vi "Parse.vi"(8 "Error In":errorcluster, 11 "object in":refnum<class "2024_5.lvclass">) -> (0 "Error Out":errorcluster, 3 "object out":refnum<class "2024_5.lvclass">)   [LabVIEW 2023, in "2024_5.lvclass"]
uses:
  2024_5.lvclass
  2024_5.lvclass/2024_5.ctl
  <vilib>/Utility/error.llb/Trim Whitespace One-Sided.vi
  <userlib>/_OpenG.lib/string/string.llb/openg_string.lvlib
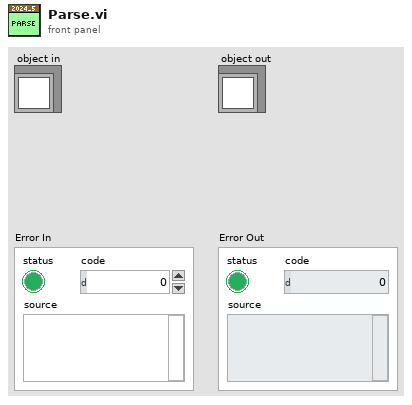
[diagram p1: front panel]
types:
  T1 = cluster{"default value 1":i64, "default value 1":i64}
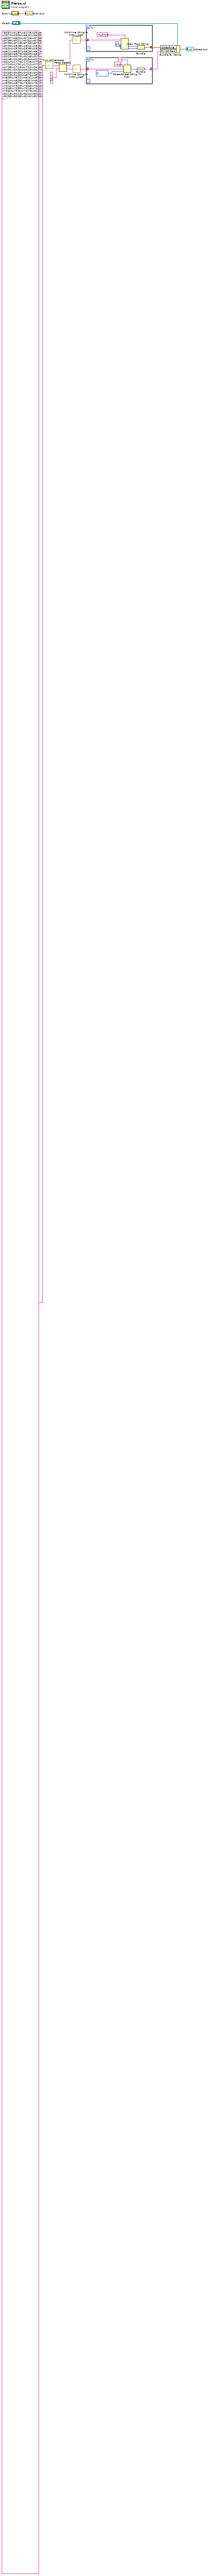
[diagram p0: block diagram]
diagram:
  n1 = call <vilib>:"Trim Whitespace.vi"("string"="39|57\n31|97\n31|75\n29|45\n29|73\n29|84\n66|91\n66|39\n66|57\n66|54\n97|16\n97|38\n97|59\n97|11\n97|62\n87|38\n87|59\n87|18\n87|93\n87|13\n87|33\n25|55\n25|22\n25|31\n25|64\n25|33\n25|85\n25|93\n68|11\n68|57\n68|36\n68|78\n68|66\n68|73\n68|39\n68|27\n32|29\n32|73\n32|45\n32|14\n32|48\n32|39\n32|54\n32|74\n32|17\n17|76\n17|45\n17|25\n17|14\n17|91\n17|11\n17|27\n17|38\n17|16\n17|22\n34|66\n34|91\n34|64\n34|29\n34|74\n34|65\n34|68\n34|26\n34|36\n34|13\n34|93\n48|76\n48|34\n48|55\n48|22\n48|42\n48|89\n48|14\n48|85\n48|87\n48|23\n48|38\n48|79\n73|62\n73|13\n73|42\n73|25\n73|55\n73|26\n73|65\n73|59\n73|18\n73|21\n73|64\n73|34\n73|79\n52|21\n52|18\n52|13\n52|22\n52|32\n52|55\n52|85\n52|42\n52|93\n52|39\n52|26\n52|66\n52|34\n52|68\n74|27\n74|57\n74|48\n74|73\n74|91\n74|16\n74|87\n74|38\n74|54\n74|75\n74|29\n74|62\n74|69\n74|84\n74|23\n38|37\n38|21\n38|13\n38|42\n38|64\n38|55\n38|66\n38|23\n38|85\n38|32\n38|79\n38|34\n38|89\n38|33\n38|52\n38|22\n69|65\n69|62\n69|38\n69|55\n69|34\n69|37\n69|33\n69|79\n69|21\n69|18\n69|87\n69|23\n69|85\n69|22\n69|16\n69|93\n69|89\n11|18\n11|85\n11|89\n11|59\n11|52\n11|22\n11|26\n11|87\n11|25\n11|76\n11|37\n11|23\n11|42\n11|21\n11|62\n11|38\n11|13\n11|69\n33|97\n33|27\n33|68\n33|29\n33|44\n33|31\n33|93\n33|66\n33|32\n33|84\n33|11\n33|45\n33|17\n33|54\n33|78\n33|75\n33|39\n33|36\n33|91\n91|79\n91|55\n91|22\n91|87\n91|23\n91|36\n91|25\n91|16\n91|76\n91|45\n91|59\n91|11\n91|75\n91|29\n91|62\n91|27\n91|69\n91|54\n91|48\n91|52\n75|34\n75|21\n75|42\n75|25\n75|76\n75|79\n75|23\n75|89\n75|18\n75|22\n75|26\n75|62\n75|69\n75|73\n75|11\n75|85\n75|37\n75|14\n75|52\n75|59\n75|38\n59|55\n59|13\n59|79\n59|32\n59|65\n59|93\n59|42\n59|52\n59|18\n59|44\n59|37\n59|85\n59|22\n59|25\n59|68\n59|33\n59|38\n59|31\n59|21\n59|23\n59|89\n59|26\n26|29\n26|39\n26|44\n26|31\n26|91\n26|17\n26|32\n26|93\n26|74\n26|66\n26|48\n26|57\n26|36\n26|97\n26|13\n26|45\n26|64\n26|65\n26|27\n26|33\n26|84\n26|78\n26|68\n79|42\n79|26\n79|57\n79|31\n79|89\n79|93\n79|18\n79|17\n79|33\n79|68\n79|74\n79|39\n79|85\n79|37\n79|78\n79|21\n79|44\n79|66\n79|65\n79|34\n79|64\n79|32\n79|97\n79|13\n42|37\n42|18\n42|13\n42|97\n42|29\n42|39\n42|78\n42|64\n42|65\n42|66\n42|89\n42|26\n42|44\n42|57\n42|85\n42|34\n42|32\n42|93\n42|31\n42|74\n42|91\n42|17\n42|33\n42|68\n18|17\n18|97\n18|44\n18|36\n18|29\n18|33\n18|91\n18|27\n18|64\n18|74\n18|57\n18|65\n18|13\n18|68\n18|84\n18|26\n18|78\n18|39\n18|66\n18|54\n18|93\n18|31\n18|32\n18|37\n22|26\n22|93\n22|13\n22|78\n22|66\n22|37\n22|31\n22|97\n22|34\n22|32\n22|85\n22|21\n22|39\n22|42\n22|65\n22|64\n22|44\n22|33\n22|89\n22|74\n22|79\n22|68\n22|55\n22|18\n62|44\n62|25\n62|85\n62|22\n62|64\n62|33\n62|13\n62|87\n62|26\n62|89\n62|16\n62|23\n62|79\n62|38\n62|59\n62|93\n62|55\n62|37\n62|18\n62|21\n62|42\n62|34\n62|65\n62|52\n21|34\n21|66\n21|93\n21|17\n21|44\n21|37\n21|68\n21|26\n21|74\n21|57\n21|18\n21|91\n21|65\n21|13\n21|31\n21|89\n21|32\n21|85\n21|39\n21|97\n21|78\n21|42\n21|64\n21|33\n93|84\n93|11\n93|57\n93|45\n93|36\n93|29\n93|76\n93|39\n93|31\n93|14\n93|91\n93|32\n93|66\n93|75\n93|48\n93|97\n93|78\n93|73\n93|74\n93|54\n93|17\n93|27\n93|44\n93|68\n23|32\n23|26\n23|68\n23|79\n23|39\n23|64\n23|25\n23|65\n23|22\n23|85\n23|31\n23|93\n23|55\n23|21\n23|13\n23|89\n23|37\n23|66\n23|52\n23|18\n23|33\n23|44\n23|42\n23|34\n84|52\n84|73\n84|11\n84|55\n84|14\n84|87\n84|76\n84|89\n84|16\n84|62\n84|48\n84|42\n84|54\n84|21\n84|69\n84|38\n84|22\n84|45\n84|79\n84|34\n84|23\n84|75\n84|59\n84|25\n16|22\n16|18\n16|85\n16|65\n16|37\n16|44\n16|13\n16|21\n16|38\n16|59\n16|25\n16|23\n16|87\n16|55\n16|68\n16|52\n16|89\n16|33\n16|34\n16|64\n16|42\n16|79\n16|26\n16|93\n85|44\n85|65\n85|39\n85|37\n85|84\n85|57\n85|64\n85|26\n85|32\n85|91\n85|74\n85|33\n85|18\n85|27\n85|78\n85|93\n85|17\n85|97\n85|66\n85|31\n85|36\n85|29\n85|13\n85|68\n55|26\n55|89\n55|64\n55|37\n55|78\n55|44\n55|93\n55|68\n55|39\n55|97\n55|79\n55|17\n55|21\n55|31\n55|85\n55|66\n55|13\n55|65\n55|42\n55|18\n55|34\n55|33\n55|32\n55|74\n65|75\n65|66\n65|11\n65|78\n65|39\n65|68\n65|44\n65|97\n65|36\n65|31\n65|45\n65|91\n65|14\n65|48\n65|33\n65|57\n65|84\n65|17\n65|93\n65|54\n65|27\n65|29\n65|74\n65|32\n76|37\n76|25\n76|42\n76|69\n76|23\n76|18\n76|16\n76|89\n76|62\n76|52\n76|34\n76|55\n76|21\n76|13\n76|79\n76|38\n76|65\n76|85\n76|26\n76|59\n76|87\n76|73\n76|64\n76|22\n27|21\n27|55\n27|38\n27|79\n27|59\n27|73\n27|75\n27|11\n27|16\n27|62\n27|42\n27|23\n27|76\n27|22\n27|45\n27|34\n27|52\n27|84\n27|87\n27|25\n27|48\n27|69\n27|54\n27|14\n14|52\n14|73\n14|22\n14|69\n14|25\n14|34\n14|16\n14|23\n14|21\n14|37\n14|38\n14|64\n14|87\n14|85\n14|59\n14|26\n14|13\n14|18\n14|76\n14|42\n14|62\n14|79\n14|55\n14|89\n36|48\n36|75\n36|23\n36|21\n36|73\n36|84\n36|54\n36|87\n36|25\n36|62\n36|42\n36|16\n36|79\n36|76\n36|27\n36|38\n36|11\n36|22\n36|69\n36|52\n36|45\n36|14\n36|55\n36|59\n13|17\n13|44\n13|27\n13|93\n13|32\n13|33\n13|66\n13|48\n13|91\n13|31\n13|54\n13|78\n13|57\n13|29\n13|64\n13|84\n13|74\n13|68\n13|39\n13|45\n13|97\n13|36\n13|75\n13|65\n57|29\n57|14\n57|54\n57|25\n57|76\n57|45\n57|59\n57|69\n57|91\n57|75\n57|87\n57|27\n57|16\n57|11\n57|22\n57|84\n57|55\n57|73\n57|38\n57|36\n57|48\n57|62\n57|52\n57|23\n89|29\n89|18\n89|66\n89|37\n89|33\n89|68\n89|39\n89|85\n89|13\n89|44\n89|97\n89|27\n89|91\n89|32\n89|93\n89|31\n89|64\n89|36\n89|74\n89|57\n89|17\n89|65\n89|26\n89|78\n78|75\n78|23\n78|45\n78|48\n78|69\n78|25\n78|17\n78|84\n78|73\n78|29\n78|36\n78|14\n78|91\n78|57\n78|76\n78|87\n78|62\n78|27\n78|38\n78|16\n78|11\n78|54\n78|59\n78|52\n64|33\n64|27\n64|44\n64|57\n64|78\n64|11\n64|65\n64|48\n64|31\n64|93\n64|39\n64|45\n64|17\n64|84\n64|91\n64|74\n64|29\n64|75\n64|68\n64|97\n64|32\n64|36\n64|54\n64|66\n54|34\n54|16\n54|79\n54|85\n54|23\n54|87\n54|69\n54|73\n54|52\n54|21\n54|14\n54|75\n54|22\n54|11\n54|48\n54|59\n54|25\n54|38\n54|45\n54|55\n54|89\n54|76\n54|62\n54|42\n37|91\n37|65\n37|44\n37|13\n37|31\n37|64\n37|17\n37|66\n37|33\n37|36\n37|78\n37|93\n37|68\n37|74\n37|32\n37|29\n37|26\n37|48\n37|39\n37|54\n37|97\n37|84\n37|57\n37|27\n44|54\n44|75\n44|68\n44|69\n44|14\n44|45\n44|97\n44|17\n44|84\n44|29\n44|74\n44|78\n44|27\n44|66\n44|31\n44|39\n44|32\n44|91\n44|57\n44|76\n44|11\n44|48\n44|73\n44|36\n45|76\n45|34\n45|73\n45|21\n45|85\n45|38\n45|59\n45|25\n45|79\n45|87\n45|11\n45|62\n45|52\n45|75\n45|16\n45|37\n45|18\n45|23\n45|22\n45|89\n45|69\n45|55\n45|42\n45|14\n39|29\n39|73\n39|48\n39|59\n39|38\n39|36\n39|87\n39|14\n39|54\n39|91\n39|17\n39|74\n39|76\n39|11\n39|62\n39|78\n39|16\n39|45\n39|69\n39|27\n39|75\n39|97\n39|84\n31|57\n31|48\n31|39\n31|11\n31|27\n31|74\n31|54\n31|66\n31|36\n31|91\n31|16\n31|78\n31|87\n31|45\n31|17\n31|76\n31|84\n31|69\n31|14\n31|29\n31|62\n31|73\n29|11\n29|87\n29|79\n29|25\n29|16\n29|36\n29|22\n29|48\n29|21\n29|62\n29|14\n29|69\n29|75\n29|55\n29|59\n29|76\n29|23\n29|52\n29|38\n29|27\n29|54\n66|14\n66|59\n66|69\n66|27\n66|75\n66|62\n66|84\n66|45\n66|17\n66|78\n66|76\n66|97\n66|87\n66|11\n66|16\n66|36\n66|73\n66|29\n66|48\n66|74\n97|27\n97|91\n97|29\n97|57\n97|78\n97|45\n97|54\n97|14\n97|48\n97|23\n97|69\n97|17\n97|36\n97|73\n97|74\n97|76\n97|84\n97|87\n97|75\n87|44\n87|85\n87|79\n87|55\n87|21\n87|23\n87|22\n87|65\n87|64\n87|42\n87|26\n87|68\n87|32\n87|52\n87|34\n87|89\n87|25\n87|37\n25|34\n25|21\n25|65\n25|42\n25|26\n25|13\n25|44\n25|79\n25|18\n25|68\n25|97\n25|89\n25|32\n25|37\n25|39\n25|74\n25|66\n68|32\n68|62\n68|45\n68|91\n68|29\n68|74\n68|54\n68|14\n68|69\n68|75\n68|84\n68|76\n68|17\n68|48\n68|97\n68|31\n32|69\n32|31\n32|11\n32|27\n32|66\n32|36\n32|97\n32|75\n32|76\n32|84\n32|91\n32|16\n32|57\n32|78\n32|62\n17|57\n17|23\n17|36\n17|69\n17|29\n17|73\n17|75\n17|62\n17|59\n17|48\n17|87\n17|84\n17|54\n17|52\n34|31\n34|57\n34|32\n34|85\n34|39\n34|37\n34|78\n34|17\n34|97\n34|44\n34|18\n34|89\n34|33\n48|52\n48|75\n48|21\n48|59\n48|18\n48|69\n48|73\n48|16\n48|62\n48|11\n48|45\n48|25\n73|52\n73|33\n73|16\n73|85\n73|89\n73|23\n73|87\n73|22\n73|38\n73|69\n73|37\n52|64\n52|31\n52|44\n52|33\n52|25\n52|97\n52|65\n52|89\n52|79\n52|37\n74|36\n74|76\n74|17\n74|11\n74|78\n74|14\n74|52\n74|45\n74|59\n38|26\n38|65\n38|31\n38|68\n38|93\n38|44\n38|25\n38|18\n69|13\n69|26\n69|25\n69|52\n69|42\n69|59\n69|64\n11|16\n11|73\n11|34\n11|55\n11|14\n11|79\n33|74\n33|14\n33|48\n33|76\n33|57\n91|14\n91|38\n91|73\n91|84\n75|55\n75|87\n75|16\n59|34\n59|64\n26|54\n\n78,45,48,38,52,62,29\n87,59,38,52,25,55,79,42,34,85,37,26,13,64,65,33,68\n57,29,84,48,45,75,11,14,76,73,69,16,38,23,22\n74,57,91,36,27,84,54,45,75,11,14,76,73,69,87,59,38\n69,62,16,87,59,38,23,52,25,22,55,79,21,42,34,89,85,18,37,26,13,64,33\n33,44,68,32,31,66,39,97,74,78,17,57,91,29,36,27,54,48,75,11,14\n32,66,39,97,74,78,17,57,91,29,36,27,84,54,48,45,11,14,73,69,62\n74,66,65,34,93,32,21,26,89,31,78,44,18,13,37,85,33,68,79,64,55\n38,52,25,55,21,34,85,18,26,13,64,33,93,44,68,32,31\n68,36,64,33,48,32,93,31,13,26,74\n48,45,75,11,76,73,69,62,87,59,38,23,22,55,79,21,42,34,85\n33,16,44,34,85,79,65,22,42,25,64,87,18,55,52,89,13\n73,69,62,16,87,59,38,23,52,25,22,55,79,21,42,89,85,18,37,26,13,64,65\n14,78,45,23,16,36,57,74,76,87,75,59,62,73,54,27,17,91,48,29,84,69,38\n33,93,44,32,31,66,97,74,78,17,57,91,29,36,84,54,48,45,75,11,14\n38,23,79,42,34,37,33,32,31\n65,93,44,68,32,31,66,39,97,74,78,17,57,91,36,27,84,54,48,75,11\n11,84,59,45,54,38,36,14,29,52,16,27,62,76,87,78,75\n54,48,45,75,11,14,76,73,69,62,16,87,59,38,23,52,25,22,55,79,21,34,89\n34,18,26,74,29,31,85,17,64\n16,87,38,52,21,34,18,37,13,64,33\n91,31,78,66,27,84,74,36,32,39,68,73,44\n69,62,36,74,45,66,54,91,14,11,27,32,75,39,84,48,73,76,31,29,17,78,97\n44,68,32,31,66,74,78,57,36,27,84,54,14,76,73\n59,73,22,21,76,62,14,23,16,79,27,36,55,75,38,54,48,11,52,45,25,84,69\n29,36,27,54,45,75,11,14,73,69,62,16,87,59,38,23,52,25,22,55,79\n64,68,39,44,93,13,31,26,74,33,22,66,79,42,55,34,18,65,89,85,37\n79,18,37,13,32,66,17\n87,38,78,57,36,62,45,17,91,59,23,84,76,75,54,14,29,27,48,16,11\n87,59,23,55,79,42,85,18,37,64,65,33,93,44,68\n68,17,57,31,11,48,54,73,14,76,91,75,69,74,78,32,84,45,97,66,29,36,39\n38,55,65,52,13,87,18,44,22,16,64,26,23,34,37,42,59,85,21\n89,85,26,13,64,65,33,68,31,66,74,17,57,91,36\n75,11,14,76,73,62,16,87,59,38,23,52,25,22,55,79,21,42,34,89,85,18,37\n59,93,33,79,62,16,55\n66,39,17,36,84,54,48,75,11\n89,21,37,79,93,25,22,52,34,42,64,55,23,68,44,65,32,66,31,26,85,18,13\n13,64,32,31,17,84,54\n16,65,25,33,55,79,21,34,87,18,64,93,52,38,37,23,59,42,62\n91,29,36,84,54,45,75,11,73,69,62,16,87,59,38,23,52,22,55\n31,66,39,17,57,27,11,62,16\n26,33,32,66,29,36,48\n18,37,26,65,33,44,32,66,39,97,57,29,36,27,84\n93,44,68,31,39,97,74,78,17,57,91,29,36,27,54,48,45,75,11,14,76\n32,31,66,39,97,78,17,57,91,29,36,27,54,48,45,75,14,76,73,69,62\n26,13,65,31,66,39,74,57,91,36,84,54,48\n68,13,32,93,85,18,25,97,39,42,34\n27,84,11,14,76,69,16,38,25\n93,66,57,27,54,75,76\n16,37,89,73,87,13,14,52,23\n85,37,26,13,65,33,93,44,32,66,39,97,17,91,29,36,27\n66,78,57,75,11,76,69\n75,11,76,73,69,62,16,87,59,38,23,52,25,22,55,79,21,42,34,89,85,18,37\n78,27,73,14,38,45,84,69,23,48,11,87,54,16,62,57,29,74,36,17,59,91,75\n33,68,17,21,39\n26,13,65,33,44,68,32,39,97,74,78,17,91,36,84,54,48\n93,13,68,34,32,37,55\n11,76,73,69,62,16,87,59,38,23,52,22,55,79,21,42,34,89,85,37,26\n14,38,23,25,79,42,89\n57,38,84,75,14,59,23\n25,34,89,18,26,13,64,65,33,93,44,31,66,39,97\n48,91,65,33,97,68,31,57,39,44,27,29,78,64,17,75,93,36,74,66,54,45,32\n87,79,13,65,33\n55,79,33,44,68,74,78\n25,52,26,65,18,13,23,22,37,59,32,42,33,85,44\n57,29,75,59,73,17,36\n16,13,89,33,21,42,65,38,55,37,59,34,44,25,85,23,22,64,87\n32,97,42,39,78,21,33,26,13,85,55\n31,84,74,91,32,78,76,36,62\n69,16,52,22,55,37,33\n13,65,33,68,32,66,39,97,74,78,17,36,27,84,54,48,45\n85,23,13,55,42,89,22,68,93,21,26,79,52,59,65,18,87,25,37,34,38\n34,75,84,23,62,54,48\n76,55,59,62,29,36,38,73,84,16,75,48,87,22,14,79,11\n93,26,21,89,64,31,78,79,17,66,13,65,33,32,44,37,68,74,34\n11,14,76,73,69,62,16,59,38,23,25,22,55,79,21,42,89,37,26\n34,85,93,32,39\n44,68,66,39,78,57,54,14,73\n42,37,21,44,85,16,64\n64,44,32,31,39,97,74,91,36,84,54,45,75\n31,66,39,74,78,17,57,91,36,27,45,75,11,14,76,73,69\n93,97,57,11,14\n65,31,57,13,78,64,45,66,17,48,68,93,54,27,29,36,32,97,44,84,39\n73,45,55,11,23,59,76,75,25,87,34,52,22\n21,34,89,85,18,37,26,13,64,65,33,93,44,68,32,31,66,39,97,74,78,17,57\n42,34,89,85,18,37,13,64,65,33,93,44,68,32,66,39,97,74,78,17,57\n18,37,79,26,11\n16,59,48,11,14,55,36,87,73,21,76,23,69,27,52,75,54,45,62,84,22\n66,78,17,57,91,36,27,84,54\n31,44,65,37,78,33,68,36,32,66,17,18,91,93,64,74,26,89,85\n89,65,79,85,22,18,64,42,55,31,34,33,97,26,13,25,68\n55,21,89,18,26,13,64,93,68,32,31,39,78\n22,18,26,44,32,31,66,39,97\n38,79,21,42,18,37,64,65,31\n34,89,85,18,26,13,64,33,93,68,66,74,78,17,57,91,29\n17,39,16,59,54,36,78,69,57,48,76,27,84,97,91,75,45,73,62,11,14\n65,33,93,44,68,32,31,74,78,17,57,91,29,36,27,84,54,48,45,75,11\n84,48,75,73,16,59,23,52,55,79,21\n93,21,32,66,55,89,42,74,85,68,22,44,13,64,26\n14,76,73,69,62,16,87,59,38,23,52,25,22,55,21,42,34,89,85,18,37,26,13\n32,74,78,27,84,45,11\n65,26,44,74,36,78,89,31,66,32,29,13,57\n89,85,26,93,68,32,31,17,57,91,29\n59,38,23,52,25,22,55,79,21,42,34,89,85,18,26,13,64,65,33,93,44,68,32\n31,66,39,74,17,91,29,36,27,84,54,48,45,75,11,76,73,62,16\n59,91,75,11,84\n91,29,36,11,69,62,16,87,25,22,55\n91,97,39,29,57,32,73,78,48,11,84,75,45,76,27,36,69,31,68,66,74,14,17\n33,93,44,85,22,26,64,31,32,65,52,66,34,55,68,39,37,42,18\n23,37,26,42,34,65,18,21,68,79,33,31,66,89,52,22,25,93,32\n55,79,89,13,32,31,78\n84,48,45,14,69,87,38\n91,29,36,27,84,54,45,75,76,73,62,87,59,38,23,52,25,22,55\n37,33,18,66,34,64,32,89,26,79,85,25,68,39,52,44,21\n76,73,87,22,79,21,26,13,64\n75,11,14,76,73,62,16,87,22,21,42,34,89,85,37\n52,25,22,55,79,21,42,34,85,18,37,26,13,65,33,93,44,68,31,66,39\n65,22,33,79,13,68,32,42,37,44,26,25,64,85,18,93,66,89,39\n73,23,34,85,37,26,65\n45,75,11,14,76,73,69,62,16,87,59,38,23,52,25,22,55,79,21,42,34,89,85\n14,59,69,87,26,13,34\n42,34,89,26,64,65,44,31,66,39,78,17,91\n18,37,26,13,93,32,31,66,97,78,57,29,36\n42,34,23,11,79,45,75,52,55,73,38,54,22,25,87\n85,34,68,65,33,21,37,26,93,89,22,79,38,52,55,44,87,42,23,13,18\n75,48,22,73,27,45,57\n14,76,73,69,16,59,38,52,22,55,79,21,34,89,18,37,13\n26,32,48,36,91,33,65,93,66\n36,39,84,13,17,57,26,32,65,54,93,37,97,78,31\n42,87,34,73,13,14,85\n66,13,37,17,91,31,57,65,27,78,84,97,68,54,39\n42,39,97,68,25,26,79,18,21,85,44,34,65,89,93,37,55,31,22\n18,34,55,37,64,44,21\n23,52,84,87,57,38,76,27,69,22,48,62,16\n26,93,29,44,54,33,31,13,66,65,84,78,64,27,74,39,37\n37,18,57,13,17,29,31,32,36,93,26\n27,87,76,29,78,48,17\n32,31,66,39,78,57,91,29,48,75,76,73,62\n59,38,55,79,21,89,85,65,33,44,32\n27,54,17,64,45,39,97,84,36,65,44,32,74\n87,38,23,52,22,21,42,34,89,37,13,65,33,93,68\n66,31,22,32,55,13,42,37,18,68,21,79,89,23,85,44,33,34,25\n93,74,39,78,17,18,64,57,13,31,33,29,36,37,84,26,32,65,27,66,97,91,44\n97,18,33,31,13,93,84,44,26\n62,73,48,27,45,54,36,97,16,84,57,76,11,69,78,91,87,59,39,29,17,74,14\n29,31,14,39,45,11,84,16,57,27,73\n66,39,29,69,87\n69,74,59,84,48,73,16,87,62,97,75,76,54,38,45,29,17,36,14,91,27\n18,64,65,33,93,44,68,32,31,66,39,97,74,78,17,57,91,29,36,27,84\n48,45,73,79,42,34,85\n75,11,76,69,62,16,87,59,23,22,55,79,21,34,85\n93,22,26,64,33,23,52,65,87,18,25,44,55,38,37,21,42,68,85,13,79,89,59\n76,69,87,59,23,52,25,79,42,34,37,13,64\n22,37,13,38,69,18,55,21,52,14,62,34,25,23,16,73,59,85,89\n79,55,62,73,85,87,26,13,69,42,76,37,64,38,16,21,23,52,25,18,59,34,22\n22,21,85,18,26,93,32,66,39,97,74\n14,57,11,17,74,29,87\n64,65,33,31,74,78,27,84,54,48,75\n85,66,68,23,21,32,93\n85,89,93,74,65,26,64,78,79,33,66,39,55\n57,29,27,54,45,11,76,16,87,59,52,25,22\n32,31,97,17,57,29,36,27,84,48,45,75,62\n69,91,76,75,14,36,97,54,11,74,62,17,29,45,27\n48,45,73,62,16,59,38,23,55,89,85\n37,26,13,65,33,93,44,68,32,31,74,78,17,91,29,27,84\n33,65,89,37,69,38,18,79,87,52,16,23,34,59,21,62,26,42,55\n74,17,91,27,84,54,48,45,75,11,14,76,73,69,62,16,87\n66,39,74,78,91,36,27,84,54,48,45,75,11,14,69,16,87\n85,25,13,55,21,64,93,38,62,79,65,23,37\n44,36,33,68,29,32,13,65,97,39,27\n16,22,38,14,62,11,52\n45,36,93,68,14,33,44,32,48\n93,57,45,97,75,78,27,76,14\n62,23,65,33,22,34,13,21,69,79,87\n22,69,14,16,52,79,73,11,37\n66,68,26,13,39,34,52,85,32,64,33\n64,33,44,68,39,74,78,17,57\n37,21,73,25,38,55,62,59,34,87,79,89,64\n84,59,73,74,75,17,91,78,23\n78,45,74,17,84,27,91,29,14\n54,45,44,27,17,39,75,31,57,64,48\n25,84,23,45,57,69,91,76,87,17,27,73,62,29,54,52,11\n97,91,29,84,45,75,11,14,76,59,38\n17,57,91,36,27,84,48,45,11,76,73,69,62,16,59,38,23,52,25\n21,42,89,85,18,37,26,13,64,65,33,44,68,32,66,39,97,74,78,17,57\n34,21,93,23,65,52,37,32,26,25,22\n21,89,87,59,16,62,26,76,55,23,11,14,25,69,42,85,79,34,38,22,37\n27,54,11,14,62,87,59,38,52,25,22,55,79\n42,34,89,85,18,37,26,13,64,65,33,93,44,68,32,31,66,39,97,74,78,17,91\n23,25,22,55,34,89,65,93,32\n68,13,38,32,18,26,93,89,52,85,22,42,44,65,25,34,21,59,33\n57,91,29,36,27,84,54,48,45,75,14,76,73,69,62,16,87,59,38,23,52,25,22\n91,29,27,14,16,52,25,22,55\n97,26,13,79,66,37,64,42,31,55,65,85,39,44,22,18,68,34,93,33,32\n87,11,17,27,36,14,29,76,75,69,78,74,59,91,38,48,62,73,16,57,23\n42,89,85,18,64,65,33,93,66,97,74,78,91\n75,11,14,76,73,69,62,16,87,59,38,23,52,25,22,55,79,21,42,34,89,18,37\n26,64,65,33,93,44,68,32,31,66,39,78,17,57,91,29,36,27,84,54,48\n38,23,22,55,42,34,89,37,26,33,93\n29,18,34,13,89,17,39,37,26\n76,73,69,62,16,87,59,38,23,52,25,22,55,79,42,34,89,85,18,37,26,13,64\n68,89,32,17,85,42,74,33,65,18,34,37,31,79,44\n23,21,73,18,42,22,34,14,79,59,69,45,25,52,87,55,75\n75,11,14,73,69,62,16,87,59,38,23,52,25,22,55,21,42,34,85,18,37\n31,26,17,39,97,36,13,65,89,29,64\n39,97,74,17,91,29,36,27,84,54,45,11,14,76,73,69,62,87,59\n65,44,32,66,97,78,57,91,36,27,54,48,45,75,11\n31,74,78,57,29,84,45,75,62\n52,25,22,55,79,21,42,34,89,85,18,37,13,65,33,44,68,32,31,66,39\n21,62,18,25,69,55,26,65,85,79,33,34,89,42,13,59,22,87,38\n91,29,27,69,38,25,55\n27,84,48,75,11,76,73,69,62,16,87,59,38,23,52,25,55,21,42\n34,32,37,55,44,52,22,42,23,26,66,85,25\n65,33,93,44,68,32,66,39,97,74,78,17,57,29,36,84,54,48,45,75,11" ("PuzzleInput")) -> ("trimmed string"=w6:string)  [unwired: 1 in]
  n2 = Match Pattern(string=w6, regular expression="\n\n") -> (before substring=w5:string, after substring=w3:string)  [unwired: 1 in, 2 out]
  n3 = call <userlib>:"Multi-line String to Array__ogtk.vi"("string"=w5) -> ("lines"=w8:string[])
  n4 = call <userlib>:"Multi-line String to Array__ogtk.vi"("string"=w3) -> ("lines"=w2:string[])
  n5 = for {
    tunnel: w8 -> [w18] mode=indexing
    tunnel: [w13] -> w4 mode=indexing
    w16 = i64 0 ("default value 1")
    n6 = Scan From String(format string="%d|%d", input string=w18, default 1=w16, default 2=w16) -> (output 1=w15:i64, output 2=w14:i64)  [unwired: 2 in, 3 out]
    n7 = Bundle("default value 1"=w15, "default value 1"=w14) -> (w13:T1)  [unwired: 1 in]
  }
  n8 = for {
    tunnel: w2 -> [w23] mode=indexing
    tunnel: [w24] -> w1 mode=indexing
    n9 = Spreadsheet String To Array(delimiter (Tab)=",", format string="%d", spreadsheet string=w23, array type (2D Dbl)=i32[] []) -> (array=w20:i32[])
    n10 = Bundle("array type (2D Dbl)"=w20) -> (w24:cluster{"array type (2D Dbl)":i32[]})  [unwired: 1 in]
  }
  n11 = Bundle By Name(cluster="object in", "OrderRule"=w4, "PrintOrders"=w1) -> (→"object out":refnum<class "2024_5.lvclass">)
  "Error Out" <- "Error In"
